vi "Standard Error Handler.vi"(8 "error in (no error)":errorcluster, 11 "source":string) -> (0 "error out":errorcluster, 3 "error?":bool)   [LabVIEW 2025]
uses:
  <vilib>/Utility/error.llb/DialogType.ctl
panel:
  out "message":string=" INSTRUCTIONS:\r\rNormal Use:  When using subVIs that incorporate the error in/error out (or error I/O) structure, place this handler where you want to inform the user of an error, typically at the end of the I/O data path, as the last action of the program.  If the error in error? is ERROR, the handler creates a message describing the error and its source.  If the type of dialog = 1 (default), the message is displayed to the user, who can only acknowedge it.  If the type = 2, the user can acknowledge the message or abort execution; aborting a program with active I/O is not recommended.  If the type = 0, no message is displayed; this is used to process the error programmatically, and the error out cluster elements are wired to individual terminals for that reason.  \r\rOther Use:\n\r\nlocal testing.  To test the error code of a subVI or function that does not have the error I/O structure, you can wire its error code and a source string to the local error code and error source inputs.  If error in error? indicates no error and error code is not equal to 0, the local code and source are substituted for the error in values, and error? is set TRUE (ERROR)."
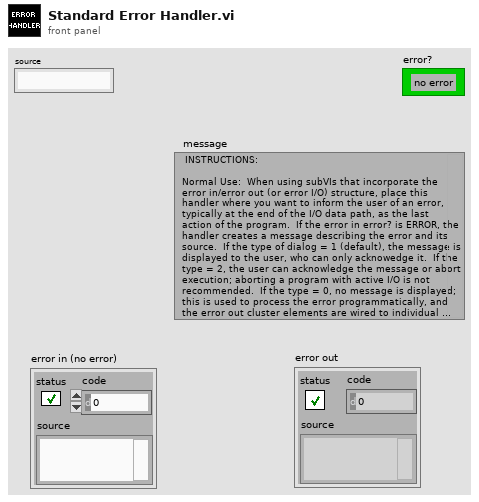
[diagram p1: front panel]
types:
  T1 = typedef "DialogType.ctl" = u16
  T2 = enum16{"open", "replace", "create", "open or create", "replace or create", "replace or create with confirmation"}
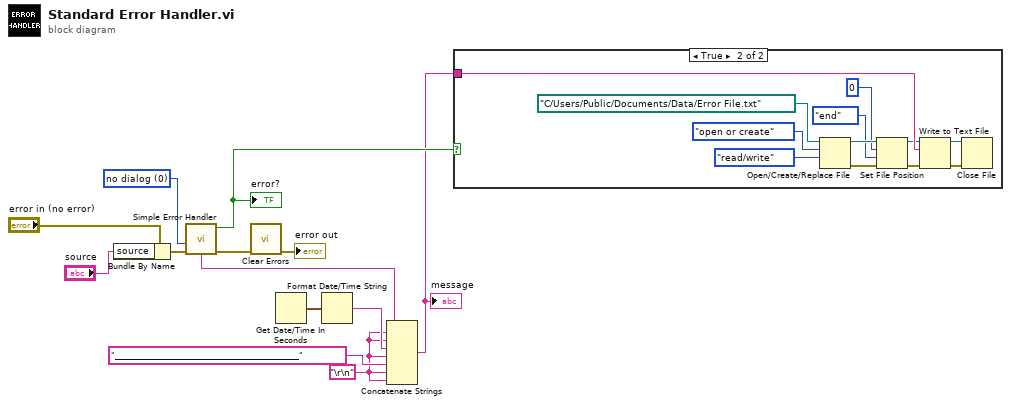
[diagram p0: block diagram]
diagram:
  w1 = "\r\n"
  w10 = T1 0 items=["no dialog", "OK message", "continue or stop message", "OK message + warnings", "continue/stop + warnings"] ("type of dialog (OK msg:1)")
  n1 = Bundle By Name(cluster="error in (no error)", "source"="source") -> (w12:errorcluster)
  n2 = call <vilib>:"Simple Error Handler.vi"("type of dialog (OK msg:1)"=w10, "error in (no error)"=w12) -> ("error?"=w4:bool, "error out"=w9:errorcluster, "message"=w6:string)  [unwired: 3 in, 2 out]
  "error?" <- w4
  n3 = call <vilib>:"Clear Errors.vi"("error in (no error)"=w9) -> ("error out"=→"error out":errorcluster)  [unwired: 5 in, 1 out]
  n4 = Get Date/Time In Seconds() -> (seconds since 1Jan1904=w7:timestamp)
  n5 = Format Date/Time String(seconds (now)=w7) -> (date/time string=w5:string)  [unwired: 2 in]
  n6 = Concatenate Strings(w6, w1, w1, w5, w1, "______________________________________________" ("string"), w1, w1) -> (w3:string)
  "message" <- w3
  n7 = case shown="True" w4 {
    tunnel: w3 -> [_ w25]
    frame False {
    }
    frame True {
      n8 = Open/Create/Replace File(file path (use dialog)=path "C:/Users/Public/Documents/Data/Error File.txt", operation (0:open)=T2."open or create", access (0:read/write)=enum16{"read/write", "read-only", "write-only"}."read/write") -> (refnum out=w19:refnum<file>, error out=w18:errorcluster)  [unwired: 3 in, 1 out]
      n9 = Set File Position(offset (in bytes) (0)=i64 0, refnum=w19, from (0:start)=enum16{"start", "end", "current"}."end", error in=w18) -> (refnum out=w16:refnum<file>, error out=w17:errorcluster)
      n10 = Write to Text File(file (use dialog)=w16, text=w25, error in=w17) -> (refnum out=w20:refnum<file>, error out=w21:errorcluster)  [unwired: 1 in, 1 out]
      n11 = Close File(refnum=w20, error in=w21) -> ()  [unwired: 2 out]
    }
  }
